vi "tdms converter.vi"() -> ()   [LabVIEW 2025]
panel:
  out "Current Repeat Progress":dbl format="%#_3g%"
  out "Current Repitition":i32
  in  "Convert":bool
  in  "Amount of repeats":i32=1 min=1 step=1
  in  "Target TDMS File":path
  in  "Source TDMS File":path
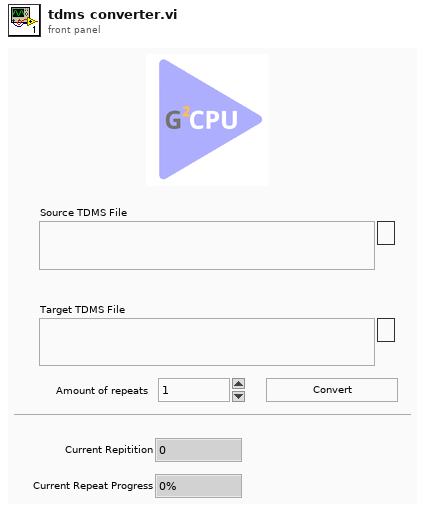
[diagram p1: front panel]
types:
  T1 = enum16{"open", "open or create", "create or replace", "create", "open (read-only)"}
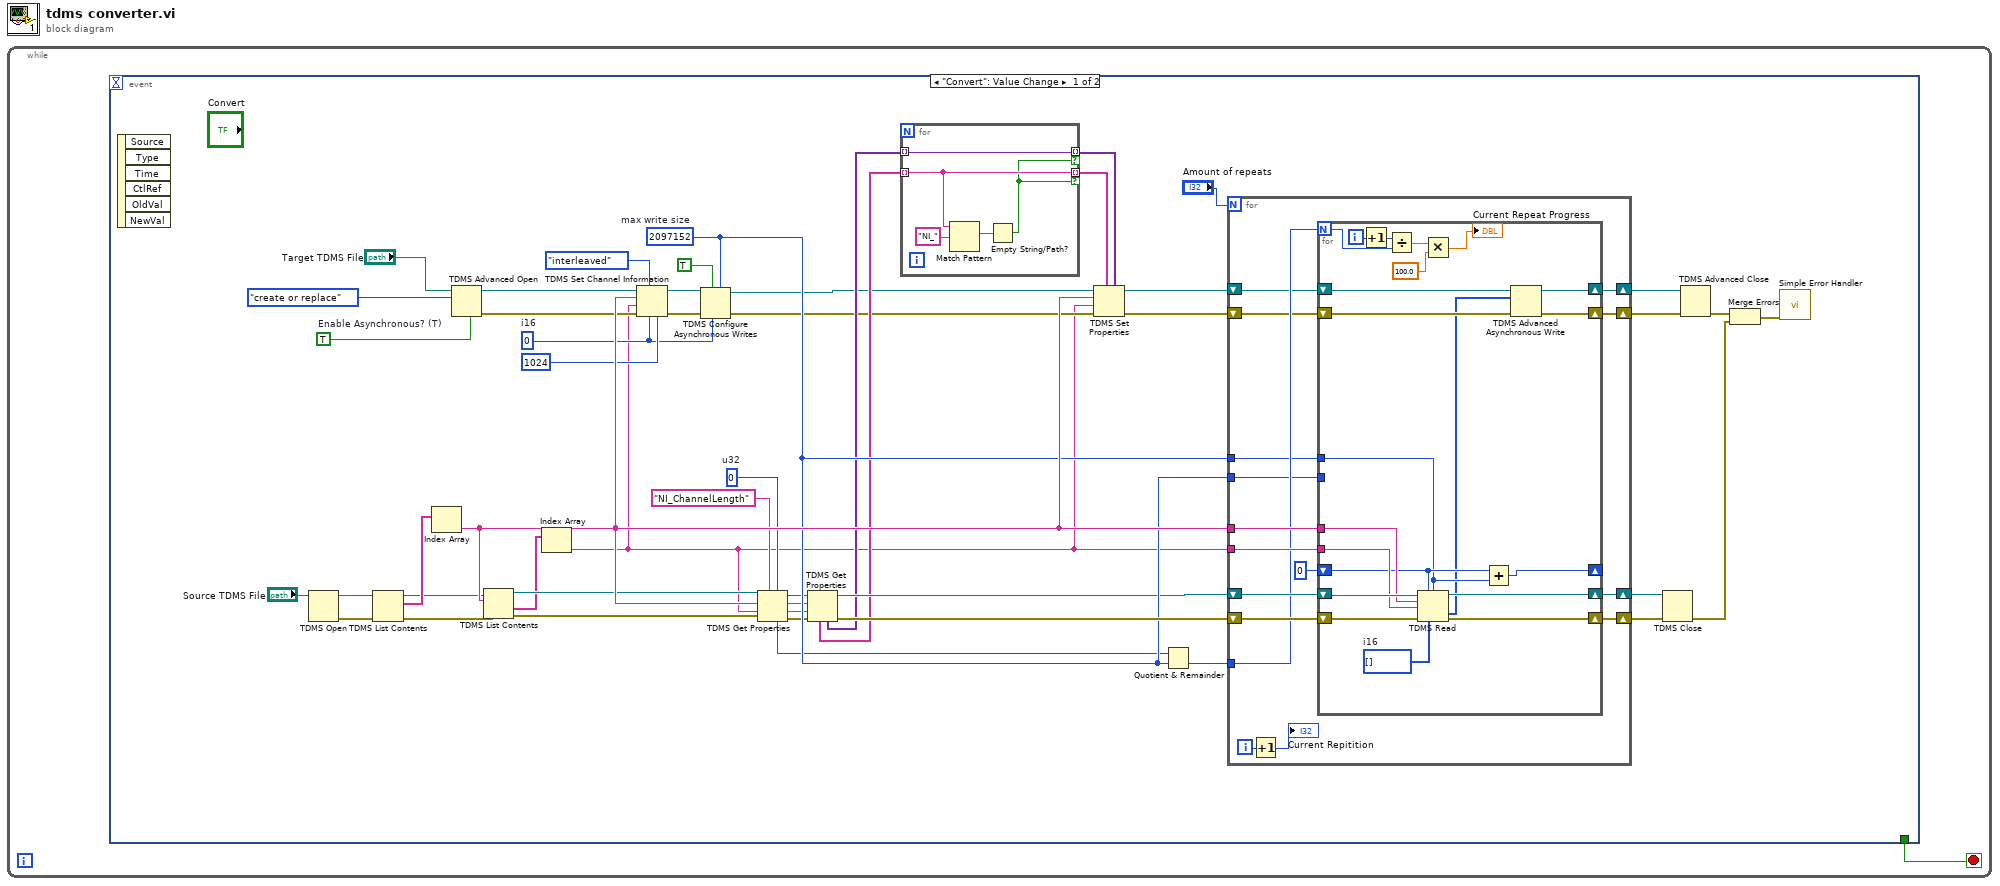
[diagram p0: block diagram]
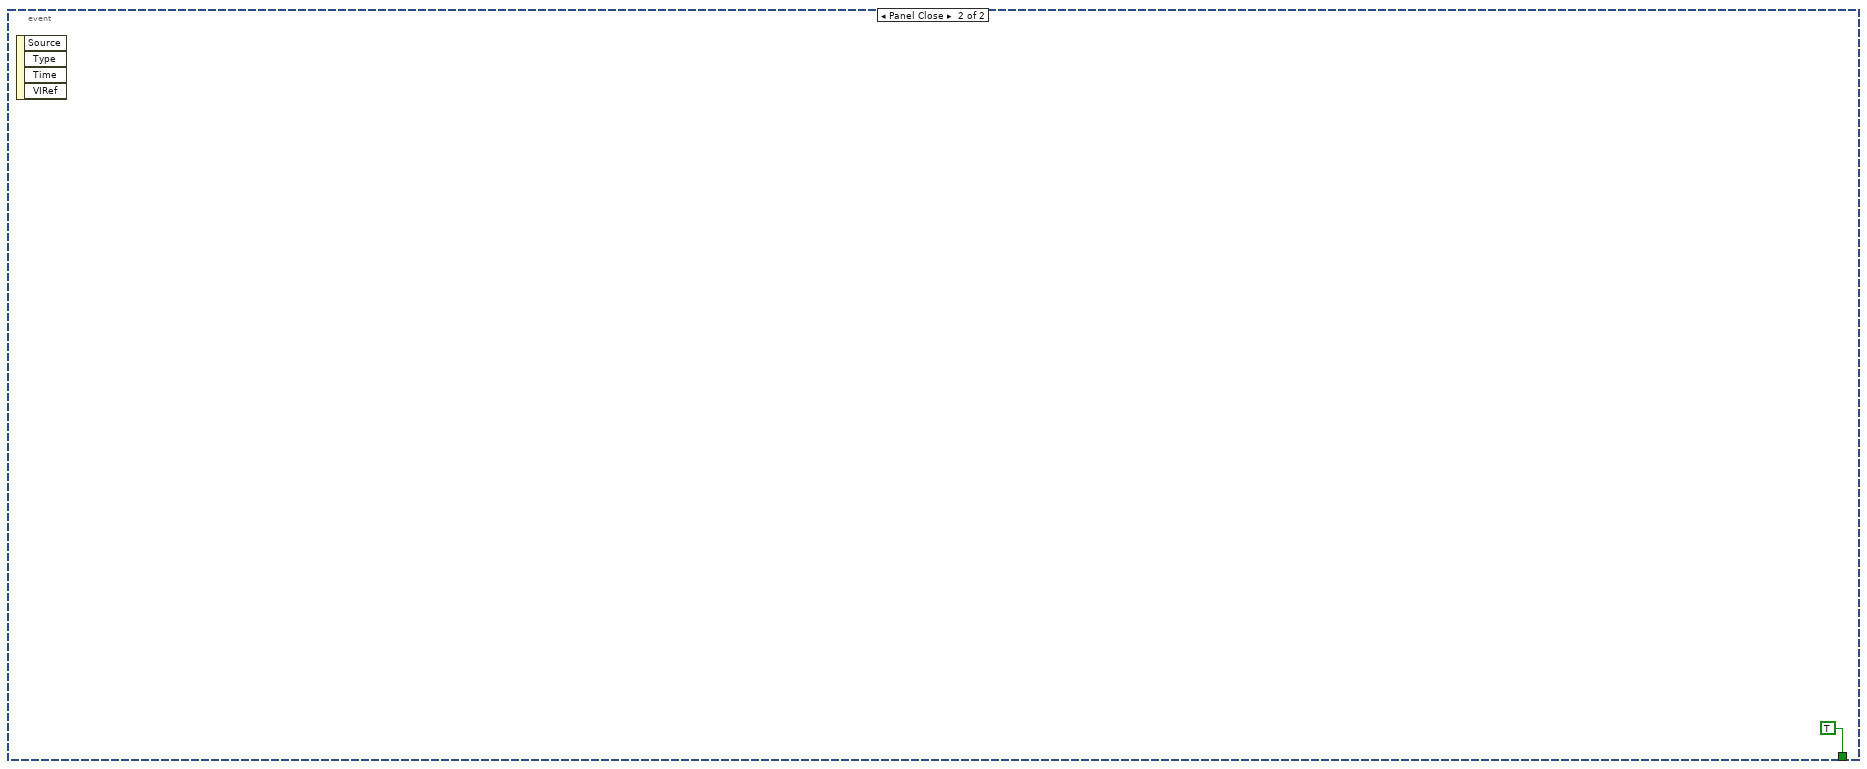
[diagram p2: hidden frame]
diagram:
  n1 = while {
    stop <- w1 stop-if-true
    n2 = event shown="[0] \"Convert\": Value Change" {
      selector: _ -> [_ _]
      dyn-events: _ -> [_ _]
      timeout: _ -> [_ _]
      tunnel: [_ TRUE] -> w1
      event "Convert": Value Change {
        w16 = u32 0  # u32
        w47 = u32 2097152  # max write size
        w17 = i16 0  # i16
        w41 = TRUE  # Enable Asynchronous? (T)
        n3 = event-data() -> ()  [unwired: 1 in, 6 out]
        n4 = TDMS Open(11:"Source TDMS File") -> (0:w34:errorcluster, 3:w35:refnum<k34>)  [unwired: 6 in]
        n5 = TDMS List Contents(4:w34, 7:w35) -> (0:w10:errorcluster, 2:w12:string[], 3:w11:refnum<k34>)  [unwired: 1 in, 1 out]
        n6 = Index Array(array=w12) -> (element=w48:string)  [unwired: 1 in]
        n7 = TDMS Advanced Open(4:w41, 10:T1."create or replace" ("operation (0:open)"), 11:"Target TDMS File") -> (0:w39:errorcluster, 3:w40:refnum<k34>)  [unwired: 2 in, 1 out]
        n8 = TDMS List Contents(4:w10, 6:w48, 7:w11) -> (0:w8:errorcluster, 1:w7:string[], 3:w9:refnum<k34>)  [unwired: 1 out]
        n9 = Index Array(array=w7) -> (element=w4:string)  [unwired: 1 in]
        n10 = TDMS Set Channel Information(4:u32 1024 ("samples per channel"), 6:w17, 7:enum16{"non-interleaved", "interleaved"}."interleaved" ("data layout (0:non-interleaved)"), 8:w39, 9:w4, 10:w48, 11:w40) -> (0:w21:errorcluster, 3:w22:refnum<k34>)
        n11 = TDMS Configure Asynchronous Writes(5:w47, 6:w17, 7:TRUE ("pre-allocate? (F)"), 8:w21, 11:w22) -> (0:w19:errorcluster, 3:w20:refnum<k34>)  [unwired: 2 in]
        n12 = TDMS Get Properties(5:w16, 7:"NI_ChannelLength" ("property name"), 8:w8, 9:w4, 10:w48, 11:w9) -> (0:w31:errorcluster, 1:w29:string, 2:w30:string, 3:w32:refnum<k34>, 4:w24:u32)  [unwired: 1 out]
        n13 = TDMS Get Properties(8:w31, 9:w29, 10:w30, 11:w32) -> (0:w49:errorcluster, 3:w28:refnum<k34>, 4:w26:variant[], 6:w27:string[])  [unwired: 2 in, 2 out]
        n14 = for {
          tunnel: w27 -> [w91] mode=indexing
          tunnel: [w92] -> w6 mode=indexing if=w88
          tunnel: w26 -> [w92] mode=indexing
          tunnel: [w91] -> w5 mode=indexing if=w88
          n15 = Match Pattern(string=w91, regular expression="NI_") -> (match substring=w89:string)  [unwired: 1 in, 3 out]
          n16 = Empty String/Path?(string/path=w89) -> (empty?=w88:bool)
        }
        n17 = TDMS Set Properties(5:w6, 7:w5, 8:w19, 9:w4, 10:w48, 11:w20) -> (0:w33:errorcluster, 3:w50:refnum<k34>)  [unwired: 2 out]
        n18 = Quotient & Remainder(x=w24, y=w47) -> (floor(x/y)=w3:u32)  [unwired: 1 out]
        n19 = for {
          N: "Amount of repeats" -> [_]
          tunnel: w48 -> [w60]
          tunnel: w4 -> [w59]
          tunnel: w3 -> [w58]
          tunnel: w47 -> [w56]
          tunnel: w47 -> [w55]
          shift-right: [w62] -> w45
          shift-left: w28 -> [w64]
          shift-right: [w61] -> w44
          shift-left: w49 -> [w63]
          shift-right: [w65] -> w46
          shift-left: w33 -> [w54]
          shift-right: [w66] -> w42
          shift-left: w50 -> [w53]
          i -> [w52]
          n20 = Increment(x=w52) -> (x+1=→"Current Repitition":i32)
          n21 = for {
            N: w58 -> [w71]
            shift-right: [w76] -> w66
            shift-left: w53 -> [w77]
            shift-right: [w75] -> w65
            shift-left: w54 -> [w74]
            shift-right: [w84] -> w62
            shift-left: w64 -> [w86]
            shift-right: [w83] -> w61
            shift-left: w63 -> [w85]
            tunnel: w60 -> [w82]
            tunnel: w59 -> [w81]
            shift-right: [w79] -> _
            shift-left: i64 0 ("offset (0)") -> [w80]
            tunnel: w56 -> [_]
            tunnel: w55 -> [w78]
            i -> [w72]
            w87 = i16[] []  # i16
            n22 = Increment(x=w72) -> (x+1=w67:i32)
            n23 = Divide(x=w67, y=w71) -> (x/y=w70:dbl)
            n24 = TDMS Read(0:w86, 1:w80, 2:w78, 5:w82, 7:w81, 11:w85, 12:w87) -> (4:w84:refnum<k34>, 10:w73:i16[], 15:w83:errorcluster)  [unwired: 1 in, 3 out]
            n25 = Multiply(x=w70, y=100.0) -> (x*y=→"Current Repeat Progress":dbl)
            n26 = Add(x=w80, y=w78) -> (x+y=w79:i64)
            n27 = TDMS Advanced Asynchronous Write(8:w74, 10:w73, 11:w77) -> (0:w75:errorcluster, 3:w76:refnum<k34>)
          }
        }
        n28 = TDMS Close(8:w44, 11:w45) -> (0:w13:errorcluster)  [unwired: 1 out]
        n29 = TDMS Advanced Close(8:w46, 11:w42) -> (0:w15:errorcluster)  [unwired: 2 in, 1 out]
        n30 = Merge Errors(w15, w13) -> (w14:errorcluster)
        n31 = call <vilib>:"Simple Error Handler.vi"("error in (no error)"=w14) -> ()  [unwired: 1 in, 8 out]
      }
      event Panel Close {
        n32 = event-data() -> ()  [unwired: 1 in, 4 out]
      }
    }
  }
